vi "Simon_game.vi"() -> ()   [LabVIEW 2025]
uses:
  <vilib>/Platform/TimedLoop/XDataNode/timing_clust.ctl
  <vilib>/Platform/TimedLoop/XDataNode/nitl_modes.ctl
  <vilib>/Platform/TimedLoop/XDataNode/wakeup.ctl
  <vilib>/numeric/Random Number (Range) I64.vi
  <vilib>/numeric/sub_Random U32.vi
  <vilib>/platform/TimedLoop/XDataNode/XDataNode.xnode
  <vilib>/Platform/TimedLoop/XDataNode/XDNodeRunTimeDep.lvlib
panel:
  out "Score":dbl
  out "String":string
  in  "Blue":bool
  in  "Yellow":bool
  in  "Red":bool
  in  "Green":bool
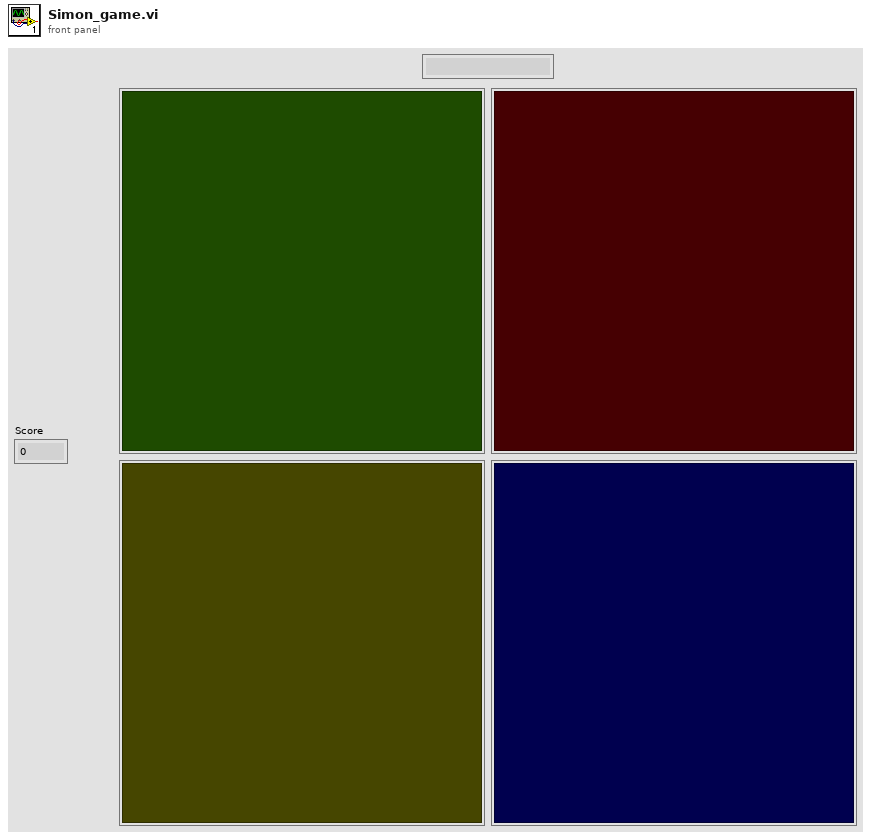
[diagram p1: front panel]
types:
  T1 = typedef "XDNodeRunTimeDep.lvlib/timing_clust.ctl" = cluster{"Expected End [f-1]":u64, "Actual End [f-1]":u64, "Finished Late? [f-1]":bool, "Expected End [i-1]":u64, "Actual End [i-1]":u64, "Finished Late? [i-1]":bool, "Expected Start [i]":u64, "Actual Start [i]":u64, "Expected Start [f]":u64, "Actual Start [f]":u64, "Source Name":string, "Structure Name":string, "Period":i64, "Deadline":i64, "Offset":i64, "Start":i64, "Priority":i32, "Timeout":i32, "Mode":T2, "Wakeup Reason":T3, "Error":errorcluster, "Source Type":string, "Secondary Source Type":string, "Global End Time":u64, "Global Start Time":u64, "Frame Duration":u64, "Iteration Duration":u64, "Assigned CPU":i32, "I/O Scan Engine Mode":u32}
  T2 = typedef "XDNodeRunTimeDep.lvlib/nitl_modes.ctl" = enum32{"No Change", "Process missed periods, maintain original phase", "Discard missed periods, maintain original phase", "Process missed periods, ignore original phase", "Discard missed periods, ignore original phase"}
  T3 = typedef "XDNodeRunTimeDep.lvlib/wakeup.ctl" = enum32{"Normal", "Aborted", "Asynchronous wakeup", "Timing source error", "Timed loop error", "Timeout"}
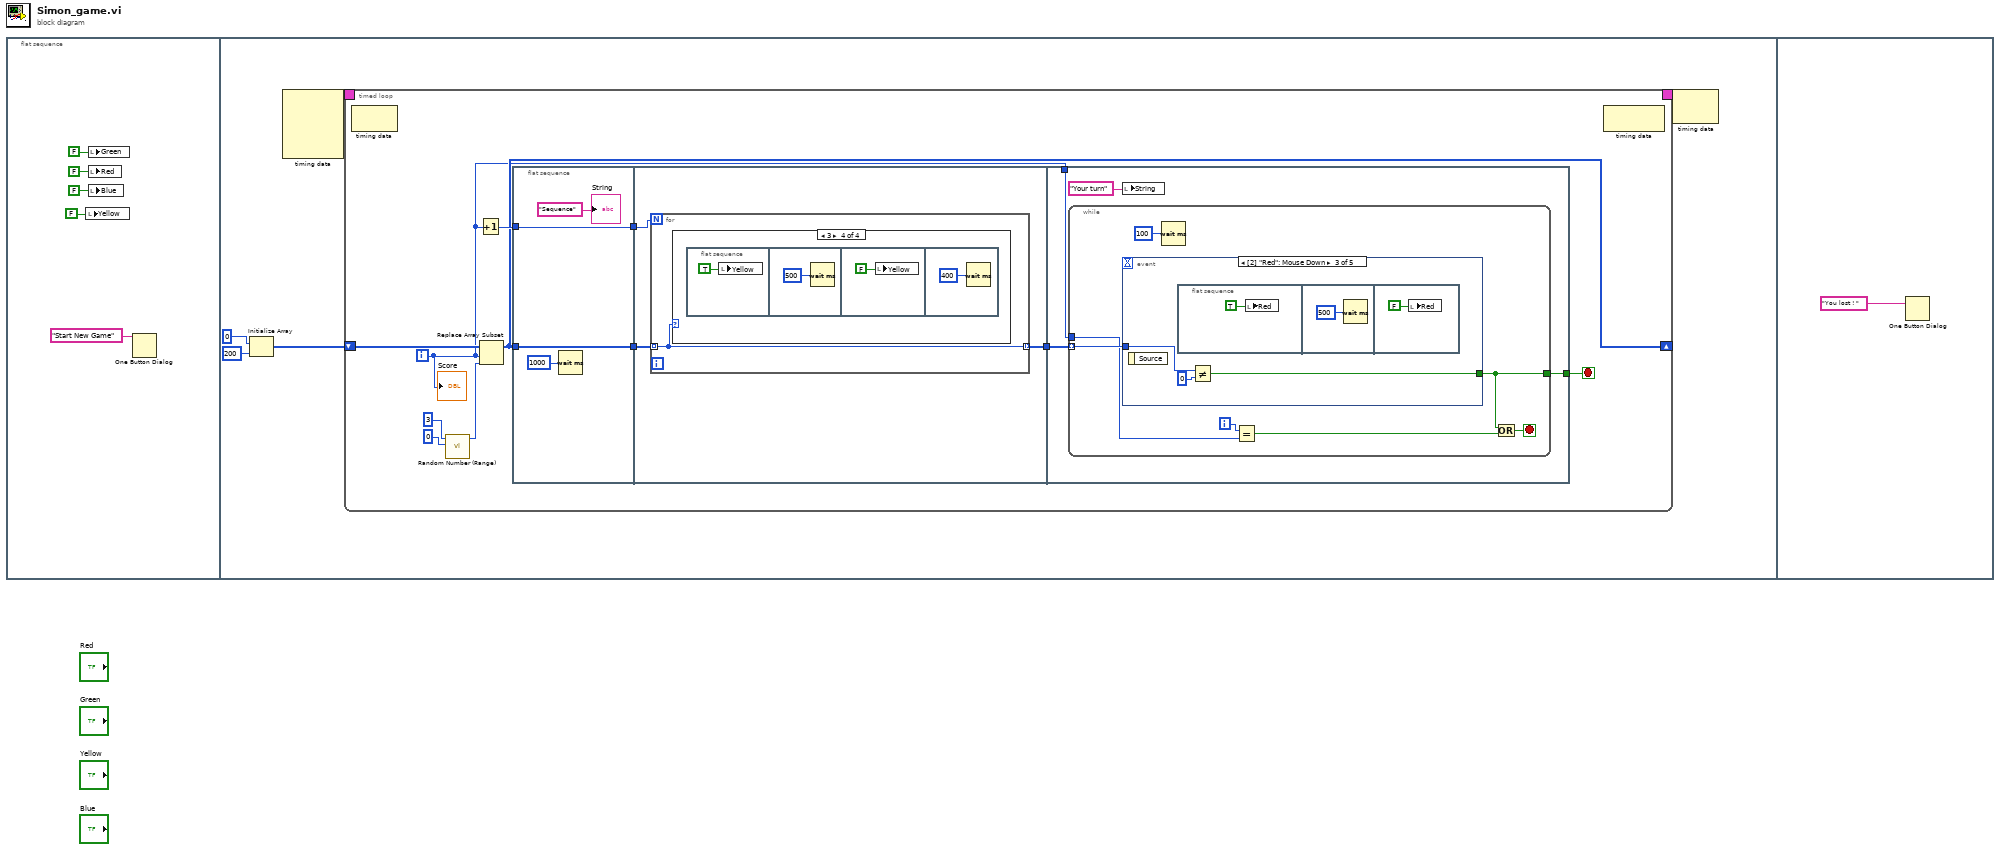
[diagram p0: block diagram]
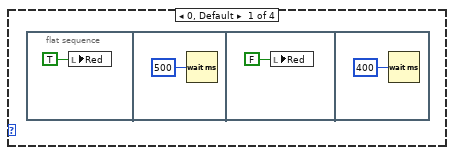
[diagram p2: hidden frame]
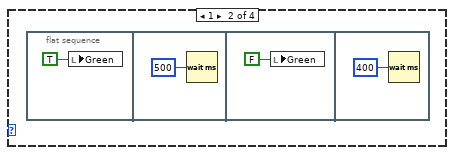
[diagram p3: hidden frame]
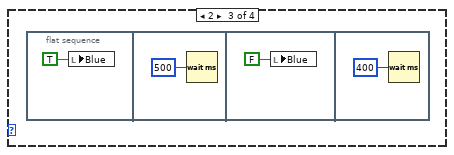
[diagram p4: hidden frame]
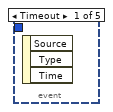
[diagram p5: hidden frame]
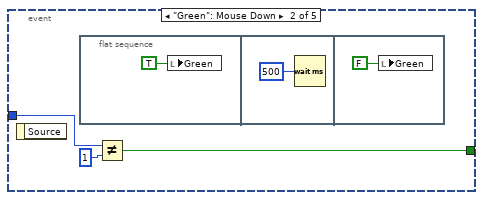
[diagram p6: hidden frame]
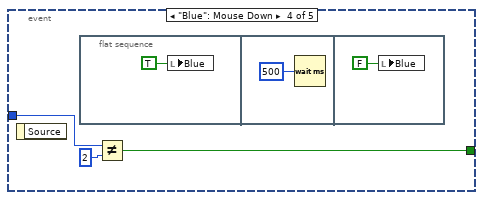
[diagram p7: hidden frame]
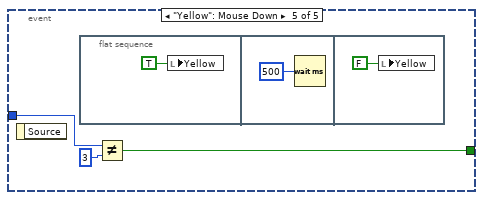
[diagram p8: hidden frame]
diagram:
  n1 = flat-sequence {
    frame #0 {
      n2 = local write "Yellow"(FALSE) -> ()
      n3 = local write "Green"(FALSE) -> ()
      n4 = local write "Red"(FALSE) -> ()
      n5 = local write "Blue"(FALSE) -> ()
      n6 = One Button Dialog(message="Start New Game" ("button name (\"OK\")")) -> ()  [unwired: 1 in, 1 out]
    }
    frame #1 {
      n7 = Initialize Array(i64 0 ("element"), 200 ("dimension size")) -> (w6:i64[])
      n8 = node-c288() -> (w10:T1)  [unwired: 4 in]
      n9 = timed-loop {
        shift-right: [w15] -> _
        shift-left: w6 -> [w17]
        timing: w10 -> [_]
        timing-out: [_] -> w9
        i -> [w11]
        stop <- w19 stop-if-true
        n10 = node-c288() -> ()  [unwired: 1 in, 1 out]
        n11 = call-poly <vilib>:"Random Number (Range).vi"("lower bound (-100)"=i64 0 ("lower bound (0)"), "upper bound (100)"=i64 3) -> ("number"=w18:i64)  [unwired: 9 in]
        n12 = Increment(x=w11) -> (x+1=w16:i32)
        n13 = Replace Array Subset(array=w17, new element=w18, index=w11) -> (w15:i64[])
        n14 = flat-sequence {
          tunnel: w16 -> [w26]
          tunnel: w15 -> [w27]
          tunnel: [w27] -> w13
          tunnel: [w26] -> w12
          tunnel: [w30] -> w14
          tunnel: w13 -> [w29]
          tunnel: w12 -> [w28]
          tunnel: w14 -> [w50]
          tunnel: [w51] -> w19
          tunnel: w11 -> [w49]
          frame #0 {
            n15 = Wait (ms)(milliseconds to wait=u32 1000) -> ()  [unwired: 1 out]
            "String" <- "Sequence" ("String")
          }
          frame #1 {
            n16 = for {
              N: w28 -> [_]
              tunnel: w29 -> [w31] mode=indexing
              tunnel: [w31] -> w30 mode=indexing
              n17 = case shown="3" w31 {
                frame 0, Default {
                  n18 = flat-sequence {
                    frame #0 {
                      n19 = local write "Red"(TRUE) -> ()
                    }
                    frame #1 {
                      n20 = Wait (ms)(milliseconds to wait=u32 500) -> ()  [unwired: 1 out]
                    }
                    frame #2 {
                      n21 = local write "Red"(FALSE) -> ()
                    }
                    frame #3 {
                      n22 = Wait (ms)(milliseconds to wait=u32 400) -> ()  [unwired: 1 out]
                    }
                  }
                }
                frame 1 {
                  n23 = flat-sequence {
                    frame #0 {
                      n24 = local write "Green"(TRUE) -> ()
                    }
                    frame #1 {
                      n25 = Wait (ms)(milliseconds to wait=u32 500) -> ()  [unwired: 1 out]
                    }
                    frame #2 {
                      n26 = local write "Green"(FALSE) -> ()
                    }
                    frame #3 {
                      n27 = Wait (ms)(milliseconds to wait=u32 400) -> ()  [unwired: 1 out]
                    }
                  }
                }
                frame 2 {
                  n28 = flat-sequence {
                    frame #0 {
                      n29 = local write "Blue"(TRUE) -> ()
                    }
                    frame #1 {
                      n30 = Wait (ms)(milliseconds to wait=u32 500) -> ()  [unwired: 1 out]
                    }
                    frame #2 {
                      n31 = local write "Blue"(FALSE) -> ()
                    }
                    frame #3 {
                      n32 = Wait (ms)(milliseconds to wait=u32 400) -> ()  [unwired: 1 out]
                    }
                  }
                }
                frame 3 {
                  n33 = flat-sequence {
                    frame #0 {
                      n34 = local write "Yellow"(TRUE) -> ()
                    }
                    frame #1 {
                      n35 = Wait (ms)(milliseconds to wait=u32 500) -> ()  [unwired: 1 out]
                    }
                    frame #2 {
                      n36 = local write "Yellow"(FALSE) -> ()
                    }
                    frame #3 {
                      n37 = Wait (ms)(milliseconds to wait=u32 400) -> ()  [unwired: 1 out]
                    }
                  }
                }
              }
            }
          }
          frame #2 {
            n38 = while {
              tunnel: w50 -> [w58] mode=indexing
              tunnel: [w56] -> w51
              tunnel: w49 -> [w53]
              i -> [w54]
              stop <- w57 stop-if-true
              n39 = event shown="[2] \"Red\": Mouse Down" {
                selector: _ -> [_ _ _ _ _]
                dyn-events: _ -> [_ _ _ _ _]
                timeout: _ -> [_ _ _ _ _]
                tunnel: w58 -> [_ w60 w67 w72 w78]
                tunnel: [_ w59 w65 w71 w77] -> w56
                event Timeout {
                  n40 = event-data() -> ()  [unwired: 1 in, 3 out]
                }
                event "Green": Mouse Down {
                  n41 = event-data() -> ()  [unwired: 1 in, 1 out]
                  n42 = flat-sequence {
                    frame #0 {
                      n43 = local write "Green"(TRUE) -> ()
                    }
                    frame #1 {
                      n44 = Wait (ms)(milliseconds to wait=u32 500) -> ()  [unwired: 1 out]
                    }
                    frame #2 {
                      n45 = local write "Green"(FALSE) -> ()
                    }
                  }
                  n46 = Not Equal?(x=w60, y=i64 1) -> (x != y?=w59:bool)
                }
                event "Red": Mouse Down {
                  n47 = event-data() -> ()  [unwired: 1 in, 1 out]
                  n48 = flat-sequence {
                    frame #0 {
                      n49 = local write "Red"(TRUE) -> ()
                    }
                    frame #1 {
                      n50 = Wait (ms)(milliseconds to wait=u32 500) -> ()  [unwired: 1 out]
                    }
                    frame #2 {
                      n51 = local write "Red"(FALSE) -> ()
                    }
                  }
                  n52 = Not Equal?(x=w67, y=i64 0) -> (x != y?=w65:bool)
                }
                event "Blue": Mouse Down {
                  n53 = event-data() -> ()  [unwired: 1 in, 1 out]
                  n54 = flat-sequence {
                    frame #0 {
                      n55 = local write "Blue"(TRUE) -> ()
                    }
                    frame #1 {
                      n56 = Wait (ms)(milliseconds to wait=u32 500) -> ()  [unwired: 1 out]
                    }
                    frame #2 {
                      n57 = local write "Blue"(FALSE) -> ()
                    }
                  }
                  n58 = Not Equal?(x=w72, y=i64 2) -> (x != y?=w71:bool)
                }
                event "Yellow": Mouse Down {
                  n59 = event-data() -> ()  [unwired: 1 in, 1 out]
                  n60 = flat-sequence {
                    frame #0 {
                      n61 = local write "Yellow"(TRUE) -> ()
                    }
                    frame #1 {
                      n62 = Wait (ms)(milliseconds to wait=u32 500) -> ()  [unwired: 1 out]
                    }
                    frame #2 {
                      n63 = local write "Yellow"(FALSE) -> ()
                    }
                  }
                  n64 = Not Equal?(x=w78, y=i64 3) -> (x != y?=w77:bool)
                }
              }
              n65 = Wait (ms)(milliseconds to wait=u32 100) -> ()  [unwired: 1 out]
              n66 = Equal?(x=w54, y=w53) -> (x = y?=w55:bool)
              n67 = Or(x=w56, y=w55) -> (x .or. y?=w57:bool)
            }
            n68 = local write "String"("Your turn" ("message")) -> ()
          }
        }
        n69 = node-c288() -> ()  [unwired: 1 in, 1 out]
        "Score" <- w11
      }
      n70 = node-c288(w9) -> ()  [unwired: 1 out]
    }
    frame #2 {
      n71 = One Button Dialog(message="You lost ! " ("button name (\"OK\")")) -> ()  [unwired: 1 in, 1 out]
    }
  }
